vi "TCP tests.vi"() -> ()   [LabVIEW 2013]
panel:
  out "bytes written":i32
  out "error out":errorcluster
  in  "remote port or service name":u16
  in  "address":string
  out "data out":string
  in  "data in":string
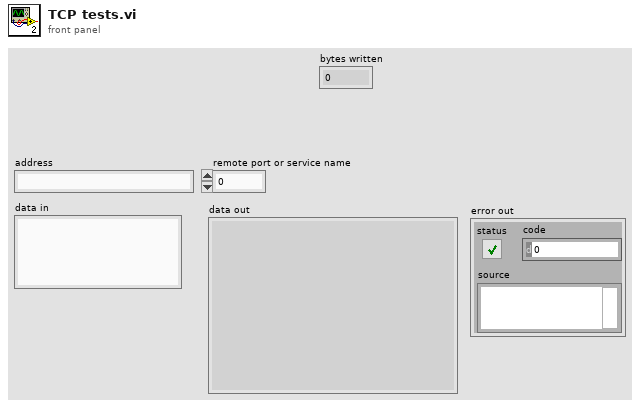
[diagram p1: front panel]
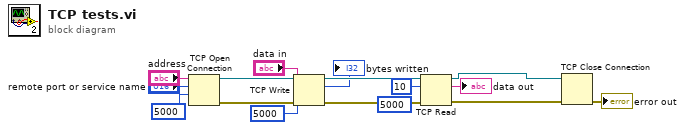
[diagram p0: block diagram]
diagram:
  n1 = TCP Open Connection(address="address", remote port or service name="remote port or service name", timeout ms (60000)=5000) -> (connection ID=w15:refnum<k5>, error out=w16:errorcluster)  [unwired: 2 in]
  n2 = TCP Write(connection ID=w15, data in="data in", error in (no error)=w16, 9:5000 ("timeout ms (25000)")) -> (connection ID out=w13:refnum<k5>, bytes written=→"bytes written":i32, error out=w14:errorcluster)
  n3 = TCP Read(connection ID=w13, bytes to read=10, error in (no error)=w14, 9:5000 ("timeout ms (25000)")) -> (connection ID out=w6:refnum<k5>, data out=→"data out":string, error out=w7:errorcluster)  [unwired: 1 in]
  n4 = TCP Close Connection(connection ID=w6, error in (no error)=w7) -> (error out=→"error out":errorcluster)  [unwired: 1 in, 1 out]
